vi "Write Solenoid Values.vi"(2 "Error In":errorcluster, 3 "LINX Resource":T1, 4 "C2 Ret Value":bool, 5 "C2 Ext Value":bool, 6 "C1 Ret Value":bool, 7 "C1 Ext Value":bool) -> (0 "Error Out":errorcluster, 1 "LINX Resource 2":T1)   [LabVIEW 2015]
uses:
  <vilib>/MakerHub/LINX/Private/Type Defs/LINX Ref.ctl
  <vilib>/MakerHub/LINX/Private/Type Defs/Platform.ctl
  <vilib>/MakerHub/LINX/Private/Type Defs/Interface.ctl
  <vilib>/MakerHub/LINX/Private/Device/Type Defs/LINX Device Config.ctl
  <vilib>/MakerHub/LINX/Private/Device/Type Defs/TCP Config.ctl
  <vilib>/MakerHub/LINX/Private/Device/Type Defs/Channels.ctl
  <vilib>/MakerHub/LINX/Public/Peripherals/Digital/Digital Write 1 Chan.vi
  <vilib>/MakerHub/LINX/LMH-LINX.lvlib
  <vilib>/MakerHub/LINX/Private/Device/Device.lvlib
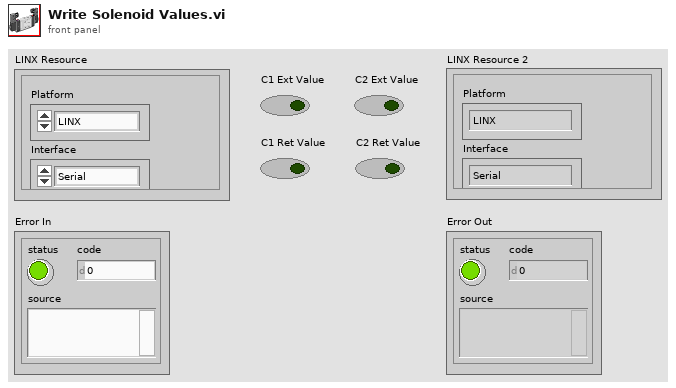
[diagram p1: front panel]
types:
  T1 = typedef "LMH-LINX.lvlib/LINX Ref.ctl" = cluster{"Platform":T2, "Interface":T3, "LINX Device Config":T4}
  T2 = typedef "LMH-LINX.lvlib/Platform.ctl" = enum16{"LINX", "myRIO"}
  T3 = typedef "LMH-LINX.lvlib/Interface.ctl" = enum16{"Serial", "TCP"}
  T4 = typedef "LMH-LINX.lvlib/Device.lvlib/LINX Device Config.ctl" = cluster{"Interface":T3, "COM Port":refnum<visa-resource-name>, "TCP Configuration":T5, "Device Family":u8, "Device ID":u8, "Device Name":string, "TCP Ref":refnum<k5>, "Channels":T6}
  T5 = typedef "LMH-LINX.lvlib/Device.lvlib/TCP Config.ctl" = cluster{"IP Address":string, "Port":u16}
  T6 = typedef "LMH-LINX.lvlib/Channels.ctl" = cluster{"DI":u8[], "DO":u8[], "AI":u8[], "AO":u8[], "PWM":u8[], "QE":u8[], "UART":u8[], "I2C 2":u8[], "SPI":u8[], "CAN":u8[], "Servo":u8[], "AI Ref (V)":dbl, "AO Ref (V)":dbl, "AO Resolution (Bits)":u8}
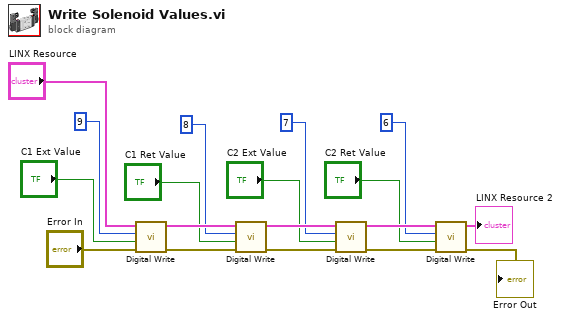
[diagram p0: block diagram]
diagram:
  n1 = call-poly <vilib>:"Digital Write.vi"("Error In"="Error In", "Output Value"="C1 Ext Value", "DO Channel"=u8 9, "LINX Resource"="LINX Resource") -> ("Error Out"=w14:errorcluster, "LINX Resource"=w15:T1)  [unwired: 6 in]
  n2 = call-poly <vilib>:"Digital Write.vi"("Error In"=w14, "Output Value"="C1 Ret Value", "DO Channel"=u8 8, "LINX Resource"=w15) -> ("Error Out"=w12:errorcluster, "LINX Resource"=w13:T1)  [unwired: 6 in]
  n3 = call-poly <vilib>:"Digital Write.vi"("Error In"=w12, "Output Value"="C2 Ext Value", "DO Channel"=u8 7, "LINX Resource"=w13) -> ("Error Out"=w10:errorcluster, "LINX Resource"=w11:T1)  [unwired: 6 in]
  n4 = call-poly <vilib>:"Digital Write.vi"("Error In"=w10, "Output Value"="C2 Ret Value", "DO Channel"=u8 6, "LINX Resource"=w11) -> ("Error Out"=→"Error Out":errorcluster, "LINX Resource"=→"LINX Resource 2":T1)  [unwired: 6 in]
